vi "FTWLib-nanomsg-Win32.vi"(11 "error in":errorcluster) -> (4 "Library Version":string, 15 "error out":errorcluster)   [LabVIEW 2013]
uses:
  FTWLib-nanomsg32.dll
panel:
  # "Inputs"
  # "Outputs"
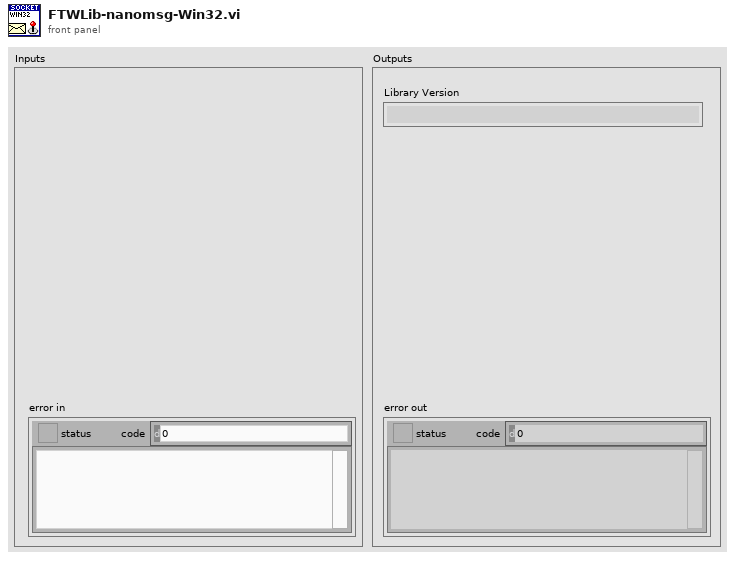
[diagram p1: front panel]
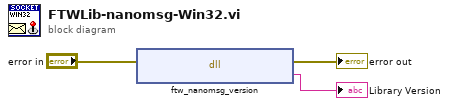
[diagram p0: block diagram]
diagram:
  n1 = dll-call lib="C:/Users/Jack/repo/ftw-master/ftw/lib/nanomsg/FTWLib-nanomsg32.dll" fn="ftw_nanomsg_version"(error in="error in") -> (error out=→"error out":errorcluster, "FTW-nanomsg Version"=→"Library Version":string)  [unwired: 2 in, 1 out]
